vi "Cluster to config string.vi"(8 "error in":errorcluster, 10 "Path":string, 11 "Cluster Ref in":refnum<vi>) -> (0 "error out":errorcluster, 2 "Config string":string, 3 "Cluster Ref out":refnum<vi>)   [LabVIEW 2012]
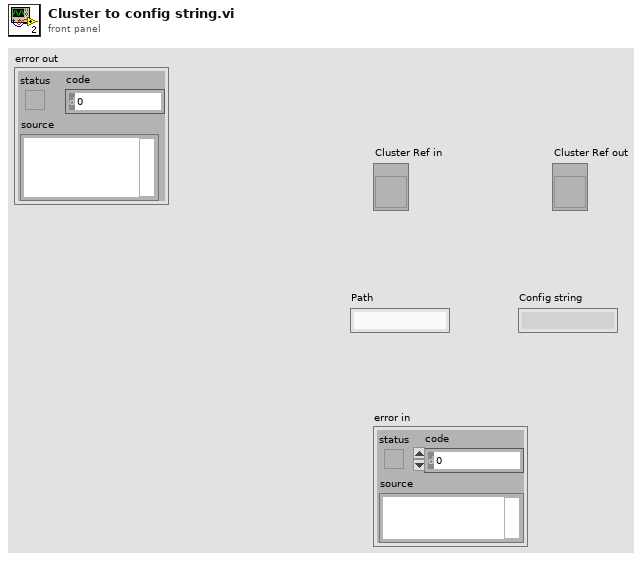
[diagram p1: front panel]
types:
  T1 = typedef "Type Enum.ctl" = enum8{"Void", "I8", "I16", "I32", "I64", "U8", "U16", "U32", "U64", "Single Float", "Double Float", "Extended Float", "Single Complex", "Double Complex", "Extended Complex", "Enum I8 NEVER", "Enum I16 NEVER", "Enum I32 NEVER", "Enum I64 NEVER", "Enum U8", "Enum U16", "Enum U32", "Enum U64", "Single Float With Unit", "Double Float With Unit", "Extended Float With Unit", "Single Complex With Unit", "Double Complex With Unit", "Extended Complex With Unit", "boolU16", "Boolean", "String", "Handle", "Path", "Picture", "C String", "Pascal String", "Tag", "SubString", "Array", "SubArray", "Cluster", "Numeric Cluster", "Variant", "LV Variant", "Measure Data (waveform)", "Refnum", "ExtData", "function", "Typedef", "Poly VI", "bad wire", "LabVIEW Class Instance"}
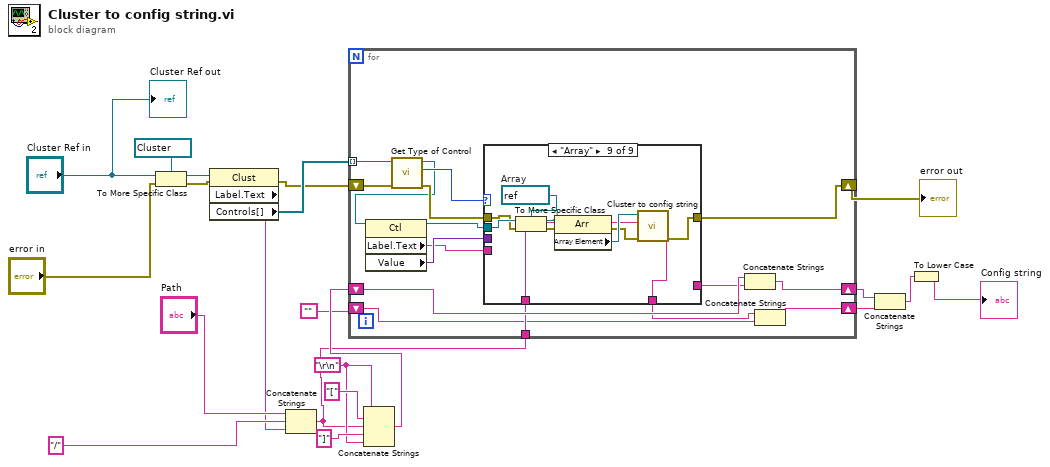
[diagram p0: block diagram]
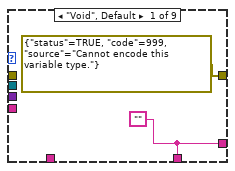
[diagram p2: hidden frame]
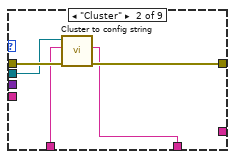
[diagram p3: hidden frame]
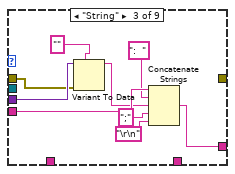
[diagram p4: hidden frame]
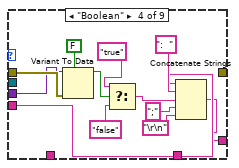
[diagram p5: hidden frame]
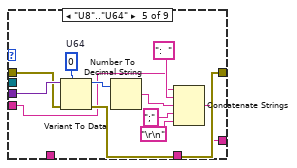
[diagram p6: hidden frame]
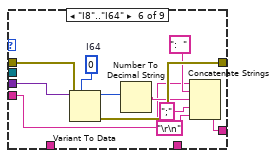
[diagram p7: hidden frame]
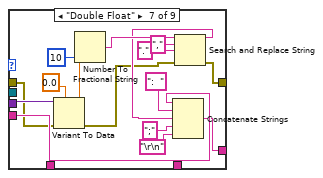
[diagram p8: hidden frame]
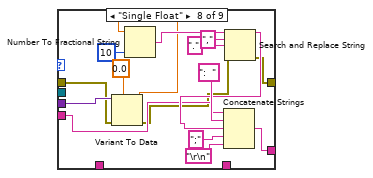
[diagram p9: hidden frame]
diagram:
  w8 = "\r\n"
  n1 = To More Specific Class(target class=refnum<vi> refnum ("reference"), reference="Cluster Ref in", error in="error in") -> (specific class reference=w19:refnum<vi>, error out=w20:errorcluster)
  n2 = property class="Clust"(reference=w19, error in=w20) -> (error out=w15:errorcluster, "Label.Text"=w11:string, "Controls[]"=w16:refnum<vi>[])  [unwired: 1 out]
  n3 = Concatenate Strings("Path", "/" ("string"), w11) -> (w6:string)
  n4 = Concatenate Strings(w8, "[", w6, "]", w8) -> (w7:string)
  n5 = for {
    tunnel: w16 -> [w37] mode=indexing
    shift-right: [w28] -> w3
    shift-left: w7 -> [w30]
    shift-right: [w27] -> w14
    shift-left: w15 -> [w35]
    tunnel: w6 -> [w26]
    shift-right: [w23] -> w2
    shift-left: "" -> [w24]
    n6 = call <vilib>:"Get Type of Control.vi"("error in (no error)"=w35, "Control Ref In"=w37) -> ("error out"=w34:errorcluster, "Type Enum"=w36:T1, "Control Ref Out"=w33:refnum<vi>)  [unwired: 7 in]
    n7 = property class="Ctl"(reference=w33) -> (reference out=w32:refnum<vi>, "Label.Text"=w25:string, "Value"=w31:variant)  [unwired: 1 in, 1 out]
    n8 = case shown="\"Array\"" w36 {
      tunnel: w34 -> [_ w44 w51 w64 w73 w84 w91 w117 w123]
      tunnel: w32 -> [_ w43 _ _ _ _ _ _ w129]
      tunnel: w31 -> [_ _ w52 w63 w74 w85 w102 w118 _]
      tunnel: w25 -> [_ _ w50 w55 w67 w78 w92 w107 _]
      tunnel: [w38 _ w45 w54 w66 w77 w88 w104 _] -> w29
      tunnel: [errorcluster {"status"=TRUE, "code"=999, "source"="Cannot encode this variable type."} ("error constant") w42 _ _ w72 w83 w89 w105 w120] -> w27
      tunnel: w26 -> [_ w41 _ _ _ _ _ _ w125]
      tunnel: [w38 w40 _ _ _ _ _ _ w124] -> w22
      frame "Void", Default {
        w38 = ""
      }
      frame "Cluster" {
        n9 = call "Cluster to config string.vi"("error in"=w44, "Path"=w41, "Cluster Ref in"=w43) -> ("error out"=w42:errorcluster, "Config string"=w40:string)  [unwired: 6 in, 1 out]
      }
      frame "String" {
        n10 = Variant To Data(error in=w51, type="" ("string"), Variant=w52) -> (data=w48:string)  [unwired: 1 out]
        n11 = Concatenate Strings(w50, ":  ", w48, ";", "\r\n") -> (w45:string)
      }
      frame "Boolean" {
        n12 = Variant To Data(error in=w64, type=FALSE, Variant=w63) -> (data=w59:bool)  [unwired: 1 out]
        n13 = Select(t="true", s=w59, f="false") -> (s? t:f=w58:string)
        n14 = Concatenate Strings(w55, ":  ", w58, ";", "\r\n") -> (w54:string)
      }
      frame "U8".."U64" {
        w76 = u64 0  # U64
        n15 = Variant To Data(error in=w73, type=w76, Variant=w74) -> (data=w75:u64, error out=w72:errorcluster)
        n16 = Number To Decimal String(number=w75) -> (decimal integer string=w68:string)  [unwired: 1 in]
        n17 = Concatenate Strings(w67, ":  ", w68, ";", "\r\n") -> (w66:string)
      }
      frame "I8".."I64" {
        w86 = i64 0  # I64
        n18 = Variant To Data(error in=w84, type=w86, Variant=w85) -> (data=w87:i64, error out=w83:errorcluster)
        n19 = Number To Decimal String(number=w87) -> (decimal integer string=w79:string)  [unwired: 1 in]
        n20 = Concatenate Strings(w78, ":  ", w79, ";", "\r\n") -> (w77:string)
      }
      frame "Double Float" {
        n21 = Variant To Data(error in=w91, type=0.0, Variant=w102) -> (data=w97:dbl, error out=w90:errorcluster)
        n22 = Number To Fractional String(number=w97, precision (6)=i16 10) -> (F-format string=w99:string)  [unwired: 2 in]
        n23 = Search and Replace String(input string=w99, search string=",", replace string="." ("replace string (\"\")"), error in=w90) -> (result string=w93:string, error out=w89:errorcluster)  [unwired: 4 in, 2 out]
        n24 = Concatenate Strings(w92, ":  ", w93, ";", "\r\n") -> (w88:string)
      }
      frame "Single Float" {
        n25 = Variant To Data(error in=w117, type=sgl 0.0, Variant=w118) -> (data=w112:sgl, error out=w106:errorcluster)
        n26 = Number To Fractional String(number=w112, precision (6)=i16 10) -> (F-format string=w115:string)  [unwired: 2 in]
        n27 = Search and Replace String(input string=w115, search string=",", replace string="." ("replace string (\"\")"), error in=w106) -> (result string=w108:string, error out=w105:errorcluster)  [unwired: 4 in, 2 out]
        n28 = Concatenate Strings(w107, ":  ", w108, ";", "\r\n") -> (w104:string)
      }
      frame "Array" {
        w128 = refnum<vi> refnum  # Array
        n29 = To More Specific Class(target class=w128, reference=w129, error in=w123) -> (specific class reference=w127:refnum<vi>, error out=w122:errorcluster)
        n30 = property class="Arr"(reference=w127, error in=w122) -> (error out=w121:errorcluster, "Array Element"=w126:refnum<vi>)  [unwired: 1 out]
        n31 = call "Cluster to config string.vi"("error in"=w121, "Path"=w125, "Cluster Ref in"=w126) -> ("error out"=w120:errorcluster, "Config string"=w124:string)  [unwired: 6 in, 1 out]
      }
    }
    n32 = Concatenate Strings(w30, w29) -> (w28:string)
    n33 = Concatenate Strings(w22, w24) -> (w23:string)
  }
  "error out" <- w14
  n34 = Concatenate Strings(w3, w2) -> (w1:string)
  n35 = To Lower Case(string=w1) -> (all lower case string=→"Config string":string)
  "Cluster Ref out" <- "Cluster Ref in"
